vi "Table Result Color.vi"(8 "Error In":errorcluster, 10 "Result Column":i32, 11 "Table Ref":refnum<vi>) -> (0 "Error Out":errorcluster)   [LabVIEW 2018]
uses:
  <vilib>/Utility/miscctls.llb/LVRowAndColumnTypeDef.ctl
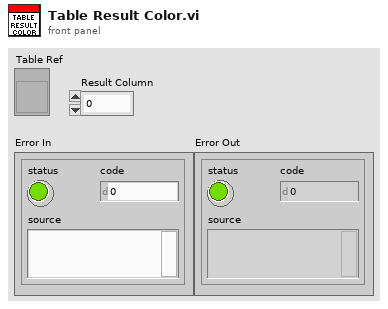
[diagram p1: front panel]
types:
  T1 = typedef "LVRowAndColumnTypeDef.ctl" = cluster{"Row":i32, "Column":i32}
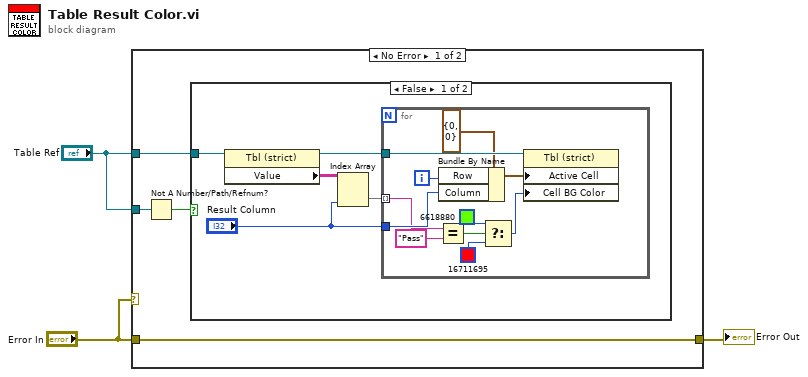
[diagram p0: block diagram]
diagram:
  n1 = case shown="No Error" "Error In" {
    tunnel: "Error In" -> [w7 w24]
    tunnel: [w7 w24] -> w2
    tunnel: "Table Ref" -> [w6 _]
    tunnel: "Table Ref" -> [w4 _]
    frame No Error {
      n2 = Not A Number/Path/Refnum?(number/path/refnum=w6) -> (NaN/Path/Refnum?=w5:bool)
      n3 = case shown="False" w5 {
        tunnel: w4 -> [w12 _]
        frame False {
          n4 = property class="Tbl (strict)"(reference=w12) -> (reference out=w9:refnum<vi>, "Value"=w11:string[][])  [unwired: 1 in, 1 out]
          n5 = Index Array(array=w11, index (col)="Result Column") -> (element=w10:string[])  [unwired: 1 in]
          n6 = for {
            tunnel: w10 -> [w18] mode=indexing
            tunnel: w9 -> [w23]
            tunnel: "Result Column" -> [w19]
            i -> [w21]
            n7 = Equal?(x=w18, y="Pass") -> (x = y?=w16:bool)
            n8 = Bundle By Name(cluster=T1 {"Row"=0, "Column"=0} ("Active Cell:Active Cell"), "Row"=w21, "Column"=w19) -> (w20:T1)
            n9 = Select(t=u32 6618880 ("Color Box"), s=w16, f=u32 16711695 ("Color Box")) -> (s? t:f=w13:u32)
            n10 = property class="Tbl (strict)"(reference=w23, "Active Cell"=w20, "Cell BG Color"=w13) -> ()  [unwired: 1 in, 2 out]
          }
        }
        frame True {
        }
      }
    }
    frame Error {
    }
  }
  "Error Out" <- w2
